vi "Stop DQMH Module.vi"(8 "Module ID":i32, 9 "Module type":T1, 10 "Module Lib":refnum<vi>, 11 "References Map":map{string, refnum<vi>}(c390)) -> (0 "error out":errorcluster)   [LabVIEW 2020, in "Panter Dashboard.lvlib"]
uses:
  Panter Dashboard.lvlib
  Module type--enum.ctl
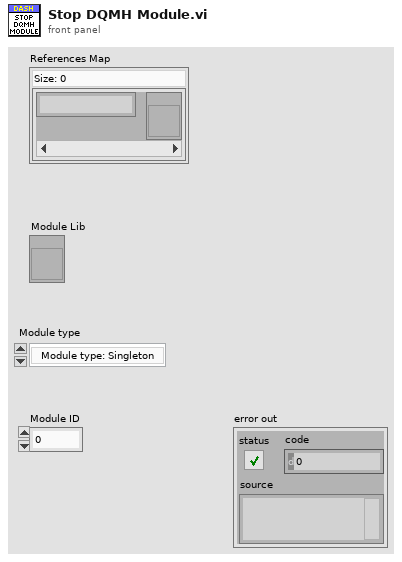
[diagram p1: front panel]
types:
  T1 = typedef "Panter Dashboard.lvlib/Module type--enum.ctl" = enum16{"Module type: Singleton", "Module type: Cloneable"}
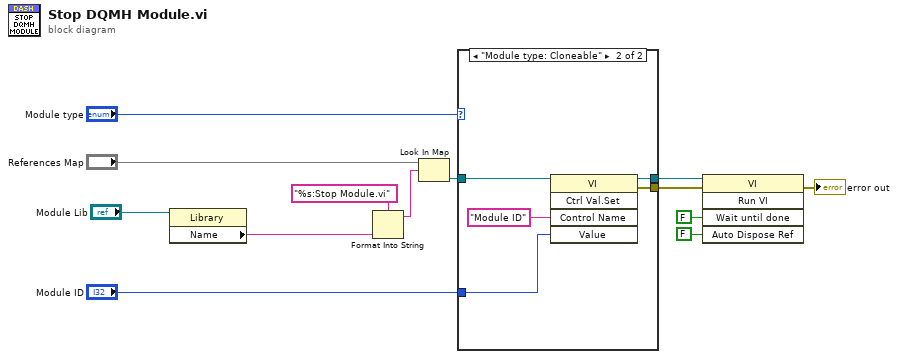
[diagram p0: block diagram]
diagram:
  n1 = property class="Library"(reference="Module Lib") -> ("Name"=w2:string)  [unwired: 1 in, 2 out]
  n2 = Format Into String(format string="%s:Stop Module.vi", w2) -> (resulting string=w8:string)  [unwired: 2 in, 1 out]
  n3 = Look In Map(map="References Map", key=w8) -> (value=w6:refnum<vi>)  [unwired: 1 in, 1 out]
  n4 = case shown="\"Module type: Cloneable\"" "Module type" {
    tunnel: [_ w19] -> w12
    tunnel: w6 -> [w14 w18]
    tunnel: "Module ID" -> [_ w17]
    tunnel: [w14 w15] -> w4
    frame "Module type: Singleton", Default {
    }
    frame "Module type: Cloneable" {
      n5 = invoke class="VI" method="Ctrl Val.Set"(reference=w18, "Control Name"="Module ID", "Value"=w17) -> (reference out=w15:refnum<vi>, error out=w19:errorcluster)  [unwired: 2 in, 3 out]
    }
  }
  n6 = invoke class="VI" method="Run VI"(reference=w4, error in=w12, "Wait until done"=FALSE ("Wait Until Done"), "Auto Dispose Ref"=FALSE ("Auto Dispose Reference")) -> (error out=→"error out":errorcluster)  [unwired: 1 in, 4 out]
